vi "_Depricated FRCts20_Backend_Event_GETFiltered.vi"(6 "Message Attributes":T4, 8 "error in (no error)":errorcluster, 10 "Data":string, 11 "Engine_Refnums":T1) -> (0 "error out":errorcluster)   [LabVIEW 2014, in "FRCts20_Backend_Engine.lvlib"]
doc: "Retrieves a specific event's data, called by the Event API. Expects an event index"
uses:
  FRCts20_Backend_Engine.lvlib
  Dependencies/Keyed Array/KeyedArray.ctl
  FRCts20_Backend_EngineRefnums.ctl
  INI_Accessor/FRCts20_Backend_INI Controller.lvclass
  Dependencies/AMC/_SubVIs/TypeDefs/Message Queue.ctl
  Dependencies/AMC/_SubVIs/TypeDefs/Message.ctl
  <vilib>/addons/database/Connection.llb/Conn ObjectReference.ctl
  FRCts20_Backend_API/FRCts20_Backend_API_Event.ctl
  FRCts20_Backend_API/FRCts20_Backend_API.lvlib
  FRCts20_Backend_FGVOperation.ctl
  FRCts20_Backend_API/FRCts20_Backend_API_SW.ctl
  Dependencies/Keyed Array/Tools_KeyedArray.lvlib
  Dependencies/AMC/AMC.lvlib
  <vilib>/addons/database/NI_Database_API.lvlib
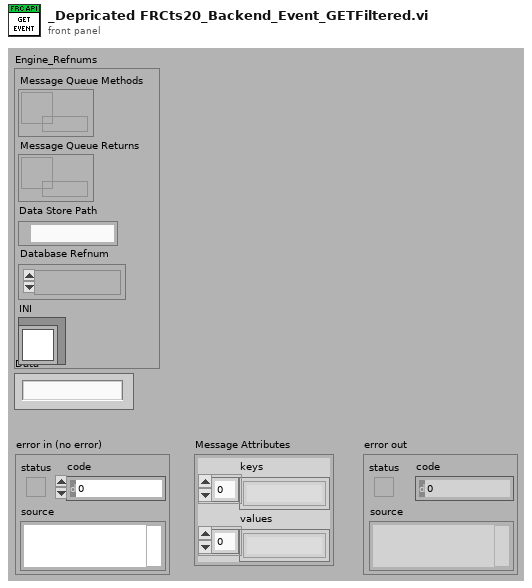
[diagram p1: front panel]
types:
  T1 = typedef "FRCts20_Backend_Engine.lvlib/FRCts20_Backend_EngineRefnums.ctl" = cluster{"Message Queue Methods":T2, "Message Queue Returns":T2, "Data Store Path":path, "Database Refnum":T3, "INI":refnum<class "FRCts20_Backend_INI Controller.lvclass">}
  T2 = typedef "AMC.lvlib/Message Queue.ctl" = refnum<queue>
  T3 = typedef "NI_Database_API.lvlib/Conn ObjectReference.ctl" = refnum<k1>
  T4 = typedef "Tools_KeyedArray.lvlib/KeyedArray.ctl" = cluster{"keys":string[], "values":string[]}
  T5 = typedef "FRCts20_Backend_Engine.lvlib/FRCts20_Backend_FGVOperation.ctl" = enum16{"Initialize", "EnqueueMessage", "EnqueueDataReturn", "FlushMessage", "FlushDataReturn"}
  T6 = typedef "FRCts20_Backend_Engine.lvlib/FRCts20_Backend_API.lvlib/FRCts20_Backend_API_Event.ctl" = cluster{"Event Index":u32, "Name":string, "Start Time":timestamp, "End Time":timestamp, "Teams":cluster{"Team Index":u32, "Team Number":u32, "Requests":cluster{"Request Number":u32, "Description":string}[], "Has Open Issue":bool}[], "SWType":T7, "APIReturn":string}
  T7 = typedef "FRCts20_Backend_Engine.lvlib/FRCts20_Backend_API.lvlib/FRCts20_Backend_API_SW.ctl" = string
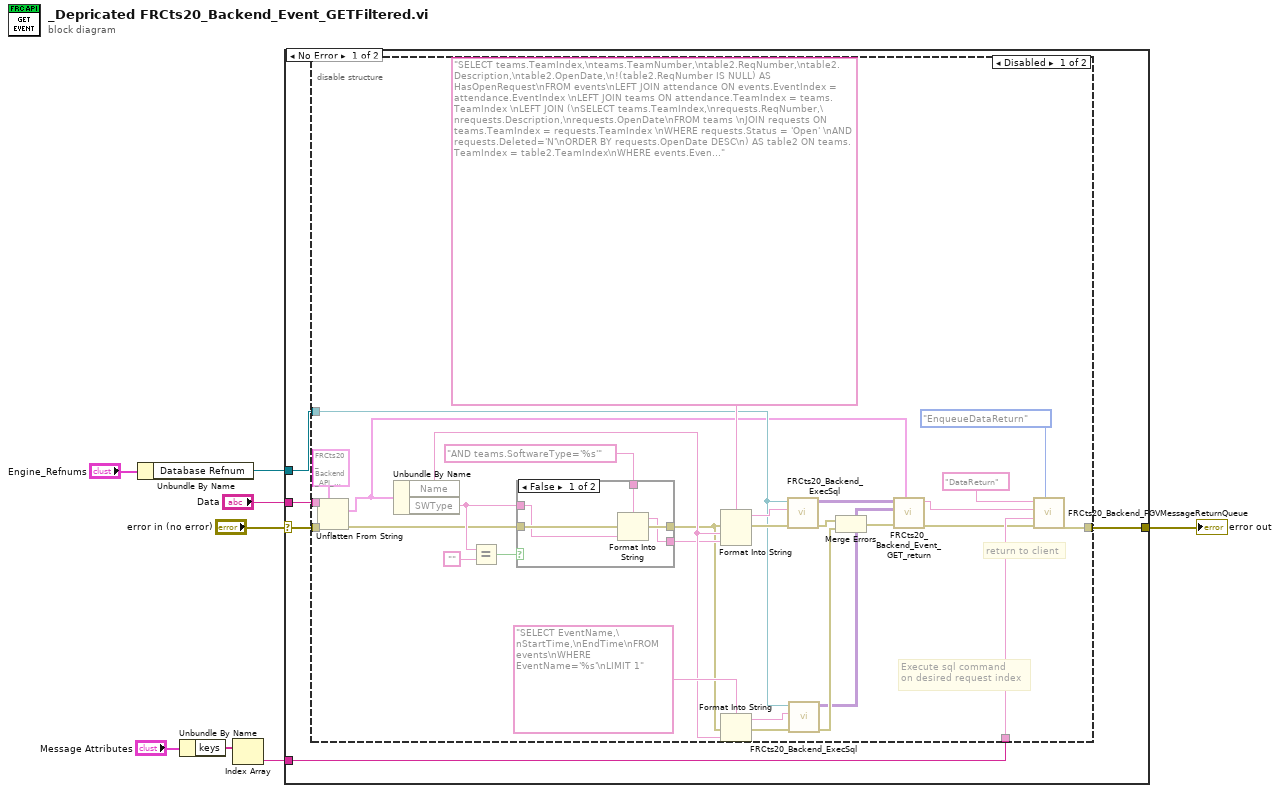
[diagram p0: block diagram]
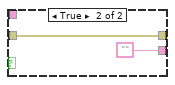
[diagram p2: hidden frame]
diagram:
  n1 = Unbundle By Name("Engine_Refnums") -> ("Database Refnum"=w1:T3)
  n2 = Unbundle By Name("Message Attributes") -> ("keys"=w4:string[])
  n3 = Index Array(array=w4) -> (element=w3:string)  [unwired: 1 in]
  n4 = case shown="No Error" "error in (no error)" {
    selector: "error in (no error)" -> [w10 w51]
    tunnel: [w13 w51] -> w7
    tunnel: w1 -> [w9 _]
    tunnel: "Data" -> [w11 _]
    tunnel: w3 -> [w12 _]
    frame No Error {
      n5 = disable-structure shown="Disabled" {
        disable-tunnel: [w43 _] -> w13
        disable-tunnel: w12 -> [w42 _]
        disable-tunnel: w11 -> [w41 _]
        disable-tunnel: w10 -> [w40 _]
        disable-tunnel: w9 -> [w27 _]
        frame Disabled {
          # "return to client"
          # "Execute sql command\non desired request index"
          n6 = Unflatten From String(type=T6 {"Event Index"=0, "Name"="", "Start Time"=timestamp(0 s since 1904-01-01), "End Time"=timestamp(0 s since 1904-01-01), "Teams"=[], "SWType"="", "APIReturn"=""} ("Competition"), binary string=w41, error in (no error)=w40) -> (value=w14:T6, error out=w18:errorcluster)  [unwired: 2 in, 1 out]
          n7 = Unbundle By Name(w14) -> ("Name"=w29:string, "SWType"=w20:T7)
          n8 = Equal?(x=w20, y="") -> (x = y?=w21:bool)
          n9 = case shown="False" w21 {
            tunnel: w20 -> [w44 _]
            tunnel: [w46 ""] -> w19
            tunnel: w18 -> [w45 w49]
            tunnel: [w47 w49] -> w17
            tunnel: "AND teams.SoftwareType='%s'" -> [w48 _]
            frame False {
              n10 = Format Into String(format string=w48, error in=w45, w44) -> (resulting string=w46:string, error out=w47:errorcluster)  [unwired: 1 in]
            }
            frame True {
            }
          }
          n11 = Format Into String(format string="SELECT teams.TeamIndex,\nteams.TeamNumber,\ntable2.ReqNumber,\ntable2.Description,\ntable2.OpenDate,\n!(table2.ReqNumber IS NULL) AS HasOpenRequest\nFROM events\nLEFT JOIN attendance ON events.EventIndex = attendance.EventIndex \nLEFT JOIN teams ON attendance.TeamIndex = teams.TeamIndex \nLEFT JOIN (\nSELECT teams.TeamIndex,\nrequests.ReqNumber,\nrequests.Description,\nrequests.OpenDate\nFROM teams \nJOIN requests ON teams.TeamIndex = requests.TeamIndex \nWHERE requests.Status = 'Open' \nAND requests.Deleted='N'\nORDER BY requests.OpenDate DESC\n) AS table2 ON teams.TeamIndex = table2.TeamIndex\nWHERE events.EventName='%s'\n%s\nORDER BY teamNumber DESC", error in=w17, w29, w19) -> (resulting string=w33:string, error out=w34:errorcluster)  [unwired: 1 in]
          n12 = Format Into String(format string="SELECT EventName,\nStartTime,\nEndTime\nFROM events\nWHERE EventName='%s'\nLIMIT 1", error in=w17, w29) -> (resulting string=w26:string, error out=w28:errorcluster)  [unwired: 1 in]
          n13 = call "FRCts20_Backend_ExecSql.vi"("error in (no error)"=w34, "format string"=w33, "Refnum in"=w27) -> ("error out"=w24:errorcluster, "recordset data"=w31:variant[][])  [unwired: 6 in, 1 out]
          n14 = call "FRCts20_Backend_ExecSql.vi"("error in (no error)"=w28, "format string"=w26, "Refnum in"=w27) -> ("error out"=w23:errorcluster, "recordset data"=w15:variant[][])  [unwired: 6 in, 1 out]
          n15 = Merge Errors(w24, w23) -> (w25:errorcluster)
          n16 = call "FRCts20_Backend_Event_GET_return.vi"("Event"=w14, "error in (no error)"=w25, 10:w15, "recordset data"=w31) -> ("error out"=w36:errorcluster, "data string"=w37:string)  [unwired: 6 in]
          n17 = call "FRCts20_Backend_FGVMessageReturnQueue.vi"("Operation"=FRCts20_Backend_FGVOperation."EnqueueDataReturn", "error in (no error)"=w36, "Key"=w42, "Message Value"=w37, "Message Name"="DataReturn") -> ("error out"=w43:errorcluster)  [unwired: 5 in, 1 out]
        }
        frame Enabled {
        }
      }
    }
    frame Error {
    }
  }
  "error out" <- w7
